vi "ButtonServoControl.vi"(7 "ServoMotorName":string="My Servo RefNum", 8 "Angle2Value":dbl, 9 "Angle1Value":dbl, 10 "Angle2Button":bool, 11 "Angle1Button":bool) -> (3 "CurrentServoAngle":u16)   [LabVIEW 2013]
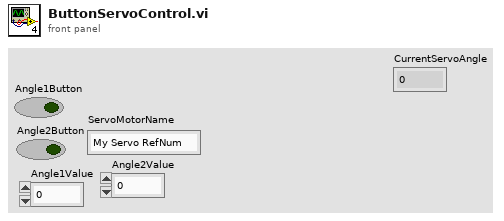
[diagram p1: front panel]
types:
  T1 = typedef "WPI_ServoDeviceRef.ctl" = cluster{"DeviceStatus":errorcluster, "Digital Module":T2, "PWM Channel":T3, "DeadBand":T4}
  T2 = typedef "FPGA_TypedefDigitalModule.ctl" = enum16{"Digital Module 1", "Digital Module 2"}
  T3 = typedef "FPGA_DIOPWMChannel.ctl" = enum8{"PWM 1", "PWM 2", "PWM 3", "PWM 4", "PWM 5", "PWM 6", "PWM 7", "PWM 8", "PWM 9", "PWM 10", "Invalid"}
  T4 = typedef "WPI_PWMDeadband.ctl" = cluster{"Name":string, "maxPositivePwm":i32, "minPositivePwm":i32, "centerPwm":i32, "maxNegativePwm":i32, "minNegativePwm":i32, "angularRange":u16}
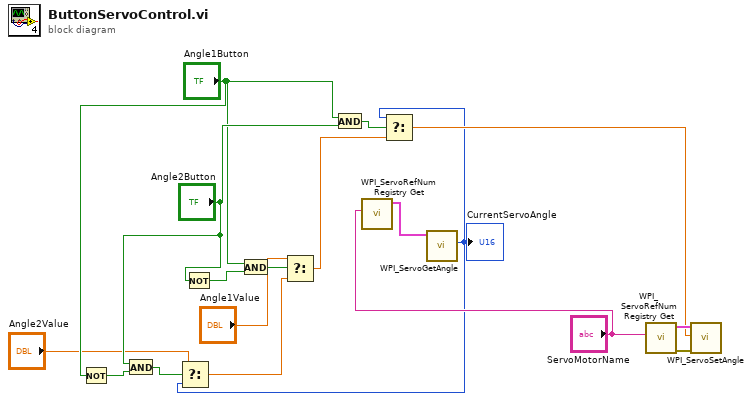
[diagram p0: block diagram]
diagram:
  n1 = Not(x="Angle1Button") -> (.not. x?=w5:bool)
  n2 = And(x="Angle2Button", y=w5) -> (x .and. y?=w6:bool)
  n3 = Not(x="Angle2Button") -> (.not. x?=w11:bool)
  n4 = And(x="Angle1Button", y=w11) -> (x .and. y?=w10:bool)
  n5 = And(x="Angle1Button", y="Angle2Button") -> (x .and. y?=w15:bool)
  n6 = call <vilib>:"WPI_ServoRefNum Registry Get.vi"("refnum name"="ServoMotorName") -> ("ServoDeviceRef"=w14:T1)  [unwired: 9 in, 1 out]
  n7 = call <vilib>:"WPI_ServoGetAngle.vi"("ServoDeviceRef"=w14) -> ("Angle"=w1:u16)  [unwired: 7 in, 2 out]
  "CurrentServoAngle" <- w1
  n8 = Select(t="Angle2Value", s=w6, f=w1) -> (s? t:f=w7:dbl)
  n9 = Select(t="Angle1Value", s=w10, f=w7) -> (s? t:f=w9:dbl)
  n10 = Select(t=w1, s=w15, f=w9) -> (s? t:f=w12:dbl)
  n11 = call <vilib>:"WPI_ServoRefNum Registry Get.vi"("refnum name"="ServoMotorName") -> ("error out"=w17:errorcluster, "ServoDeviceRef"=w16:T1)  [unwired: 9 in]
  n12 = call <vilib>:"WPI_ServoSetAngle.vi"("error in (no error)"=w17, "Angle"=w12, "ServoDeviceRef"=w16) -> ()  [unwired: 7 in, 2 out]
